vi "LoadImages.vi"(8 "error in (no error)":errorcluster, 9 "Sim Image Index":i32, 10 "Images":T1[](array[typedef]), 11 "Folder Simulation Images":path) -> (0 "error out":errorcluster, 2 "scan number":string, 3 "shot number":string)   [LabVIEW 2020, in "MagSpec_Bella.lvclass"]
uses:
  MagSpec_Bella.lvclass
  <vilib>/vision/Image Controls.llb/IMAQ Image.ctl
  <userlib>/_OpenG.lib/array/array.llb/Remove Duplicates from 1D Array (String)__ogtk.vi
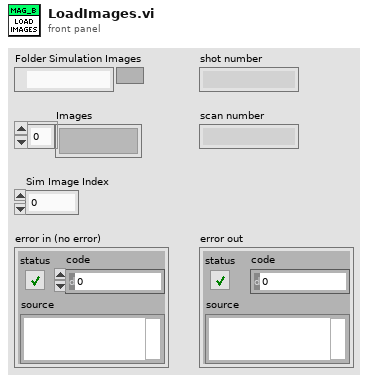
[diagram p1: front panel]
types:
  T1 = typedef "IMAQ Image.ctl" = refnum<image>
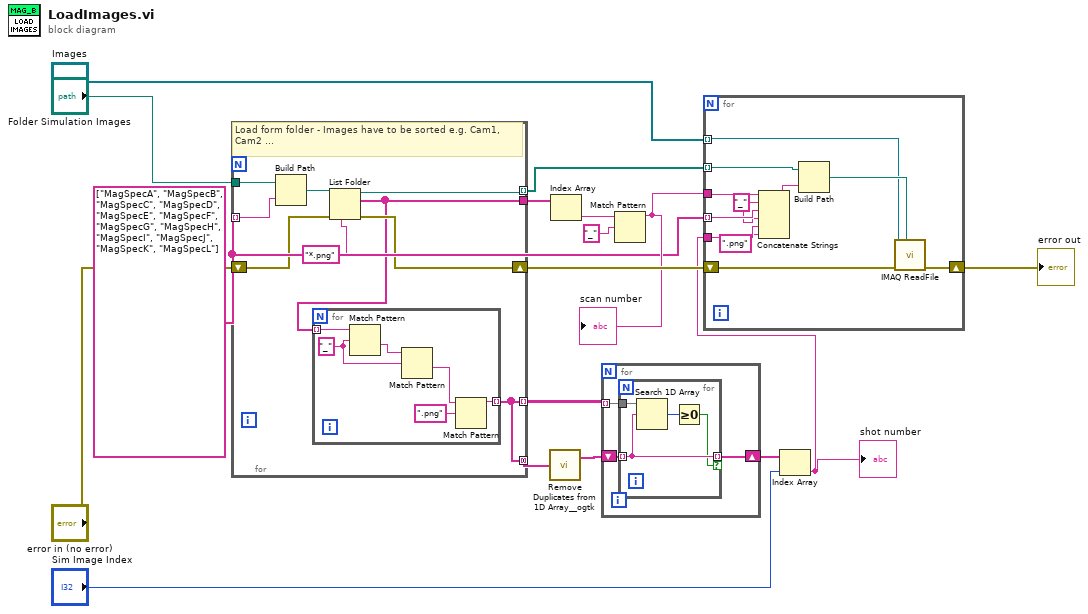
[diagram p0: block diagram]
diagram:
  w10 = string[] ["MagSpecA", "MagSpecB", "MagSpecC", "MagSpecD", "MagSpecE", "MagSpecF", "MagSpecG", "MagSpecH", "MagSpecI", "MagSpecJ", "MagSpecK", "MagSpecL"]
  n1 = for {
    tunnel: "Folder Simulation Images" -> [w26]
    shift-right: [w22] -> w17
    shift-left: "error in (no error)" -> [w23]
    tunnel: w10 -> [w25] mode=indexing
    tunnel: [w20] -> w5
    tunnel: [w19] -> w3 mode=indexing
    tunnel: [w19] -> w2 mode=concatenating
    tunnel: [w18] -> w11 mode=indexing
    # "Load form folder - Images have to be sorted e.g. Cam1, Cam2 ..."
    n2 = Build Path(base path=w26, name or relative path=w25) -> (appended path=w24:path)
    n3 = List Folder(path=w24, pattern="*.png", error in=w23) -> (path out=w18:path, filenames=w20:string[], error out=w22:errorcluster)  [unwired: 1 in, 1 out]
    n4 = for {
      tunnel: w20 -> [w32] mode=indexing
      tunnel: [w27] -> w19 mode=indexing
      w30 = "_" ("regular expression")
      n5 = Match Pattern(string=w32, regular expression=w30) -> (after substring=w31:string)  [unwired: 1 in, 3 out]
      n6 = Match Pattern(string=w31, regular expression=w30) -> (after substring=w29:string)  [unwired: 1 in, 3 out]
      n7 = Match Pattern(string=w29, regular expression=".png") -> (before substring=w27:string)  [unwired: 1 in, 3 out]
    }
  }
  n8 = call-poly <userlib>:"Remove Duplicates from 1D Array__ogtk.vi"("Input Array"=w2) -> ("Output Array"=w4:string[])  [unwired: 1 out]
  n9 = Index Array(array=w5) -> (element=w7:string)  [unwired: 1 in]
  n10 = for {
    tunnel: w3 -> [w35] mode=indexing
    shift-right: [w33] -> w8
    shift-left: w4 -> [w34]
    n11 = for {
      tunnel: w35 -> [w39]
      tunnel: w34 -> [w37] mode=indexing
      tunnel: [w37] -> w33 mode=indexing if=w36
      n12 = Search 1D Array(1D array=w39, element=w37) -> (index of element=w38:i32)  [unwired: 1 in]
      n13 = Greater Or Equal To 0?(x=w38) -> (x >= 0?=w36:bool)
    }
  }
  n14 = Match Pattern(string=w7, regular expression="_") -> (before substring=w15:string)  [unwired: 1 in, 3 out]
  "scan number" <- w15
  n15 = Index Array(array=w8, index="Sim Image Index") -> (element=w16:string)
  "shot number" <- w16
  n16 = for {
    tunnel: w15 -> [w50]
    tunnel: w10 -> [w49] mode=indexing
    tunnel: w16 -> [w47]
    tunnel: w11 -> [w44] mode=indexing
    tunnel: "Images" -> [w42] mode=indexing
    shift-right: [w41] -> w13
    shift-left: w17 -> [w40]
    w48 = "_" ("string")
    n17 = Concatenate Strings(w50, w48, w49, w48, w47, ".png" ("string")) -> (w45:string)
    n18 = Build Path(base path=w44, name or relative path=w45) -> (appended path=w43:path)
    n19 = call "IMAQ ReadFile"("File Path"=w43, "error in (no error)"=w40, "Image"=w42) -> ("error out"=w41:errorcluster)  [unwired: 4 in, 4 out]
  }
  "error out" <- w13
